vi "Resolve.vi"(7 "GlobalThreshold":T1=enum."INFO", 8 "error in (no error)":errorcluster, 9 "HostApplicationPath":path, 10 "ConfigFilePath":path, 11 "DefaultFileAppenderConfig":T2={"common"={"id"="", "threshold"=enum."INFO", "filter"={"mode"=enum."Mirror", "levelMin"=enum."INFO", "levelMax"=enum."INFO", "tagPrefix"=""}, "queueBound"=0, "dropPolicy"=enum."DropOldest", "useUTC"=FALSE}, "file"={"rootFolder"=path "", "maxFileSize"=0, "maxFileCount"=0, "baseName"="", "extension"="", "delimiter"="", "calendarFolderTree"=FALSE}}) -> (0 "error out":errorcluster, 3 "ResolvedConfig":T8={"schemaVersion"="", "globalThreshold"=enum."INFO", "defaultFileAppender"={"common"={"id"="", "threshold"=enum."INFO", "filter"={"mode"=enum."Mirror", "levelMin"=enum."INFO", "levelMax"=enum."INFO", "tagPrefix"=""}, "queueBound"=0, "dropPolicy"=enum."DropOldest", "useUTC"=FALSE}, "file"={"rootFolder"=path "", "maxFileSize"=0, "maxFileCount"=0, "baseName"="", "extension"="", "delimiter"="", "calendarFolderTree"=FALSE}}})   [LabVIEW 2026, in "Lumberjack.lvlib"]
uses:
  Lumberjack.lvlib
  TypeDefs/ConfigDTO/FilterDTO.ctl
  TypeDefs/ConfigDTO/AppenderConfigDTO.ctl
  TypeDefs/ConfigDTO/FileAppenderConfigDTO.ctl
  TypeDefs/ConfigDTO/LumberjackConfigDTO.ctl
  TypeDefs/Severity.ctl
  TypeDefs/FilterMode.ctl
  TypeDefs/Filter.ctl
  TypeDefs/DropPolicy.ctl
  TypeDefs/AppenderConfig.ctl
  TypeDefs/FileAppenderConfig.ctl
  TypeDefs/LumberjackConfig.ctl
  TypeDefs/ConfigDTO/FileConfigDTO.ctl
  TypeDefs/FileConfig.ctl
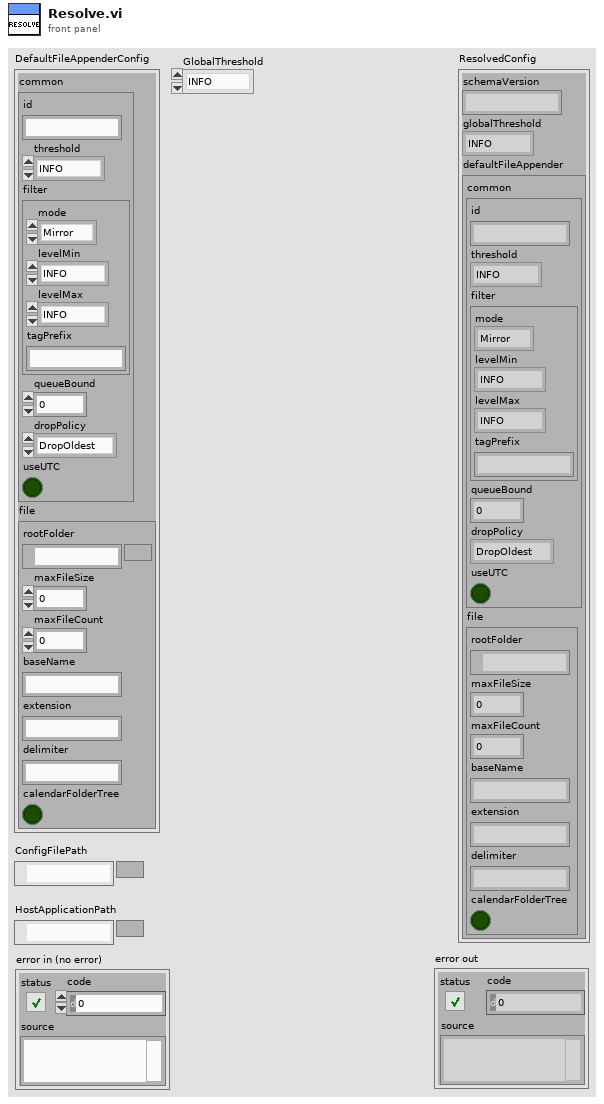
[diagram p1: front panel]
types:
  T1 = typedef "Lumberjack.lvlib/Severity.ctl" = enum16{"OFF", "FATAL", "ERROR", "WARN", "INFO", "DEBUG", "TRACE", "ALL"}
  T2 = typedef "Lumberjack.lvlib/FileAppenderConfig.ctl" = cluster{"common":T3, "file":T7}
  T3 = typedef "Lumberjack.lvlib/AppenderConfig.ctl" = cluster{"id":string, "threshold":T1, "filter":T4, "queueBound":i32, "dropPolicy":T6, "useUTC":bool}
  T4 = typedef "Lumberjack.lvlib/Filter.ctl" = cluster{"mode":T5, "levelMin":T1, "levelMax":T1, "tagPrefix":string}
  T5 = typedef "Lumberjack.lvlib/FilterMode.ctl" = enum16{"Mirror", "Routed"}
  T6 = typedef "Lumberjack.lvlib/DropPolicy.ctl" = enum16{"DropOldest", "DropNewest", "LevelAware"}
  T7 = typedef "Lumberjack.lvlib/FileConfig.ctl" = cluster{"rootFolder":path, "maxFileSize":i64, "maxFileCount":i32, "baseName":string, "extension":string, "delimiter":string, "calendarFolderTree":bool}
  T8 = typedef "Lumberjack.lvlib/LumberjackConfig.ctl" = cluster{"schemaVersion":string, "globalThreshold":T1, "defaultFileAppender":T2}
  T9 = typedef "Lumberjack.lvlib/LumberjackConfigDTO.ctl" = cluster{"schemaVersion":string, "globalThreshold":string, "defaultFileAppender":T10}
  T10 = typedef "Lumberjack.lvlib/FileAppenderConfigDTO.ctl" = cluster{"common":T11, "file":T13}
  T11 = typedef "Lumberjack.lvlib/AppenderConfigDTO.ctl" = cluster{"id":string, "threshold":string, "filter":T12, "queueBound":i32, "dropPolicy":string, "useUTC":bool}
  T12 = typedef "Lumberjack.lvlib/FilterDTO.ctl" = cluster{"mode":string, "levelMin":string, "levelMax":string, "tagPrefix":string}
  T13 = typedef "Lumberjack.lvlib/FileConfigDTO.ctl" = cluster{"rootFolder":string, "maxFileSize":i64, "maxFileCount":i32, "baseName":string, "extension":string, "delimiter":string, "calendarFolderTree":bool}
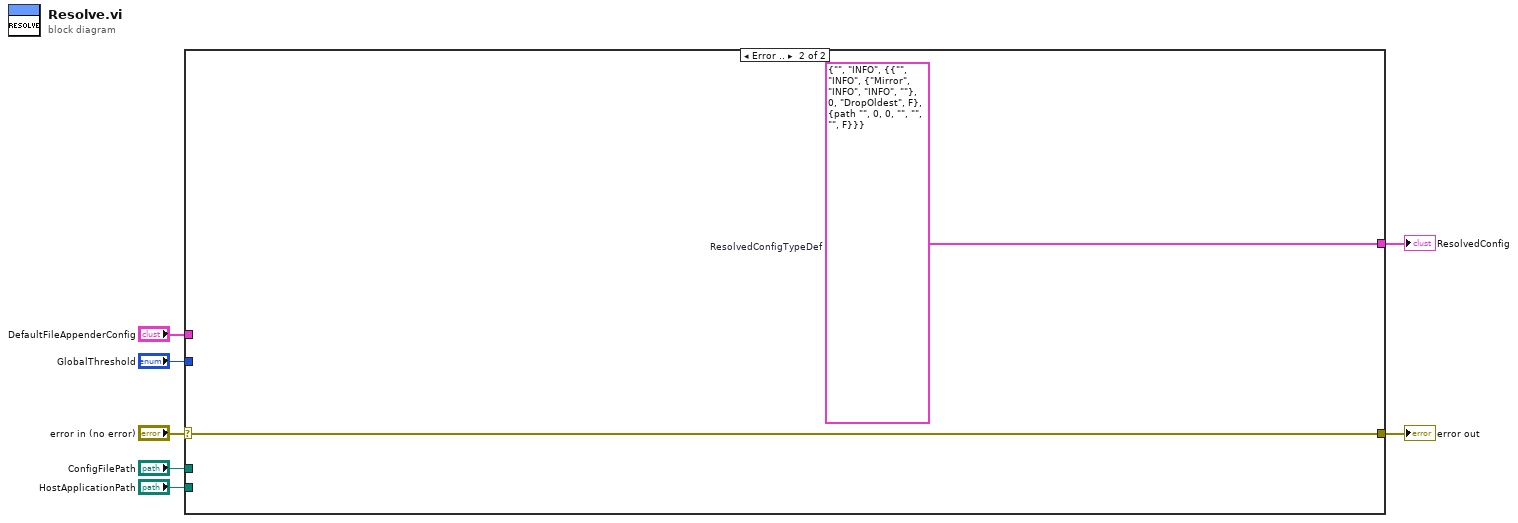
[diagram p0: block diagram]
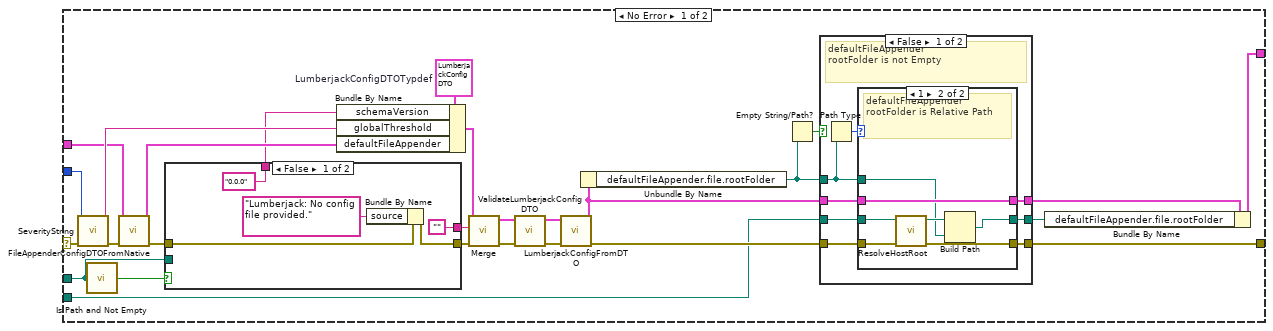
[diagram p2: hidden frame]
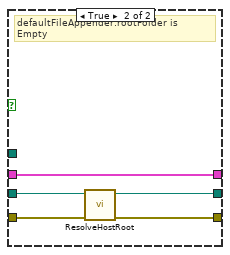
[diagram p4: hidden frame]
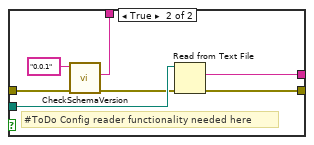
[diagram p5: hidden frame]
diagram:
  n1 = case shown="Error .." "error in (no error)" {
    selector: "error in (no error)" -> [w9 w71]
    tunnel: [w10 w71] -> w6
    tunnel: "GlobalThreshold" -> [w34 _]
    tunnel: "DefaultFileAppenderConfig" -> [w26 _]
    tunnel: "ConfigFilePath" -> [w18 _]
    tunnel: "HostApplicationPath" -> [w17 _]
    tunnel: [w11 w70] -> w1
    frame No Error {
      w33 = T9 {"schemaVersion"="", "globalThreshold"="INFO", "defaultFileAppender"={"common"={"id"="", "threshold"="INFO", "filter"={"mode"="mirror", "levelMin"="INFO", "levelMax"="INFO", "tagPrefix"=""}, "queueBound"=0, "dropPolicy"="dropOldest", "useUTC"=FALSE}, "file"={"rootFolder"="", "maxFileSize"=0, "maxFileCount"=0, "baseName"="", "extension"="", "delimiter"="", "calendarFolderTree"=FALSE}}}  # LumberjackConfigDTOTypdef
      n2 = call "SeverityString.vi"("error in (no error)"=w9, "Severity"=w34) -> ("error out"=w24:errorcluster, "SeverityString"=w32:string)  [unwired: 8 in]
      n3 = call <vilib>:"Is Path and Not Empty.vi"("path"=w18) -> ("Is Path and Not Empty?"=w27:bool)  [unwired: 4 in]
      n4 = call "FileAppenderConfigDTOFromNative.vi"("error in (no error)"=w24, "FileAppenderConfig"=w26) -> ("error out"=w23:errorcluster, "FileAppenderConfigDTO"=w25:T10)  [unwired: 8 in]
      n5 = case shown="False" w27 {
        tunnel: w23 -> [w62 w64]
        tunnel: w18 -> [_ w69]
        tunnel: [w61 w68] -> w29
        tunnel: ["" w67] -> w28
        tunnel: ["0.0.0" ("CurrentSchemaVersion") w66] -> w8
        frame False {
          n6 = Bundle By Name(cluster=w62, "source"="Lumberjack: No config file provided.") -> (w61:errorcluster)
        }
        frame True {
          # "#ToDo Config reader functionality needed here"
          n7 = call "CheckSchemaVersion.vi"("error in (no error)"=w64, "schemaVersionIn"="0.0.1") -> ("error out"=w65:errorcluster, "CurrentSchemaVersion"=w66:string)  [unwired: 7 in, 1 out]
          n8 = Read from Text File(file (use dialog)=w69, error in=w65) -> (text=w67:string, error out=w68:errorcluster)  [unwired: 2 in, 2 out]
        }
      }
      n9 = Bundle By Name(cluster=w33, "schemaVersion"=w8, "globalThreshold"=w32, "defaultFileAppender"=w25) -> (w20:T9)
      n10 = call "Merge.vi"("error in (no error)"=w29, "JSONText"=w28, "BaselineDTO"=w20) -> ("error out"=w31:errorcluster, "MergedDTO"=w30:T9)  [unwired: 7 in]
      n11 = call "ValidateLumberjackConfigDTO.vi"("error in (no error)"=w31, "BaselineDTO"=w30) -> ("error out"=w22:errorcluster, "MergedDTO"=w21:T9)  [unwired: 8 in]
      n12 = call "LumberjackConfigFromDTO.vi"("error in (no error)"=w22, "LumberjackConfigDTO"=w21) -> ("error out"=w19:errorcluster, "LumberjackConfig"=w16:T8)  [unwired: 8 in]
      n13 = Unbundle By Name(w16) -> ("defaultFileAppender.file.rootFolder"=w15:path)
      n14 = Empty String/Path?(string/path=w15) -> (empty?=w14:bool)
      n15 = case shown="False" w14 {
        tunnel: w19 -> [w42 w57]
        tunnel: w17 -> [w41 w56]
        tunnel: w16 -> [w39 w53]
        tunnel: w15 -> [w36 _]
        tunnel: [w38 w53] -> w13
        tunnel: [w37 w54] -> w10
        tunnel: [w35 w55] -> w12
        frame False {
          # "defaultFileAppender\nrootFolder is not Empty"
          n16 = Path Type(1:w36) -> (0:w40:i16)
          n17 = case shown="1" w40 {
            tunnel: w42 -> [w44 w52]
            tunnel: w41 -> [_ w51]
            tunnel: w39 -> [w45 w50]
            tunnel: [w45 w50] -> w38
            tunnel: [w44 w49] -> w37
            tunnel: w36 -> [w43 w47]
            tunnel: [w43 w46] -> w35
            frame 0, Default {
              # "defaultFileAppender\nrootFolder is Absolute Path"
            }
            frame 1 {
              # "defaultFileAppender  rootFolder is Relative Path"
              n18 = call "ResolveHostRoot.vi"("error in (no error)"=w52, "HostApplicationPath"=w51) -> ("error out"=w49:errorcluster, "HostRoot"=w48:path)  [unwired: 8 in]
              n19 = Build Path(base path=w48, name or relative path=w47) -> (appended path=w46:path)
            }
          }
        }
        frame True {
          # "defaultFileAppender.rootFolder is  Empty"
          n20 = call "ResolveHostRoot.vi"("error in (no error)"=w57, "HostApplicationPath"=w56) -> ("error out"=w54:errorcluster, "HostRoot"=w55:path)  [unwired: 8 in]
        }
      }
      n21 = Bundle By Name(cluster=w13, "defaultFileAppender.file.rootFolder"=w12) -> (w11:T8)
    }
    frame Error {
      w70 = T8 {"schemaVersion"="", "globalThreshold"=enum."INFO", "defaultFileAppender"={"common"={"id"="", "threshold"=enum."INFO", "filter"={"mode"=enum."Mirror", "levelMin"=enum."INFO", "levelMax"=enum."INFO", "tagPrefix"=""}, "queueBound"=0, "dropPolicy"=enum."DropOldest", "useUTC"=FALSE}, "file"={"rootFolder"=path "", "maxFileSize"=0, "maxFileCount"=0, "baseName"="", "extension"="", "delimiter"="", "calendarFolderTree"=FALSE}}}  # ResolvedConfigTypeDef
    }
  }
  "error out" <- w6
  "ResolvedConfig" <- w1
